vi "Init Module.vi"(8 "error in (no error)":errorcluster, 11 "Singleton Module Admin in":refnum<class "Delacor_lib_QMH_Module Admin.lvclass">) -> (0 "error out":errorcluster, 2 "DBModule Request Events":T1, 3 "Singleton Module Admin out":refnum<class "Delacor_lib_QMH_Module Admin.lvclass">)   [LabVIEW 2022 SP3, in "DBModule.lvlib"]
doc: "Initialize the module by creating Broadcast Events, Request Events, and synchronization rendezvous.\n____\nHAMPEL SOFTWARE ENGINEERING v2.6.0 (2023-12-19 10:54)"
uses:
  DBModule.lvlib
  <vilib>/Delacor/Delacor QMH/Libraries/Module Admin_class/Delacor_lib_QMH_Module Admin.lvclass
  Request Events--cluster.ctl
  Stop Argument--cluster.ctl
  Show Panel Argument--cluster.ctl
  Hide Panel Argument--cluster.ctl
  Get Module Execution Status Argument--cluster.ctl
  Show Diagram Argument--cluster.ctl
  Configure Argument--cluster.ctl
  Prepare Argument--cluster.ctl
  Request UI Display Argument--cluster.ctl
  Libraries/hse-libraries/Source/hse-dqmh/Controls/Module Display Scenarios.ctl
  Request UI Display (Reply Payload)--cluster.ctl
  Start and Configure DB_Connector Argument--cluster.ctl
  Libraries/hse-libraries/Source/hse-dqmh/hse-dqmh.lvlib
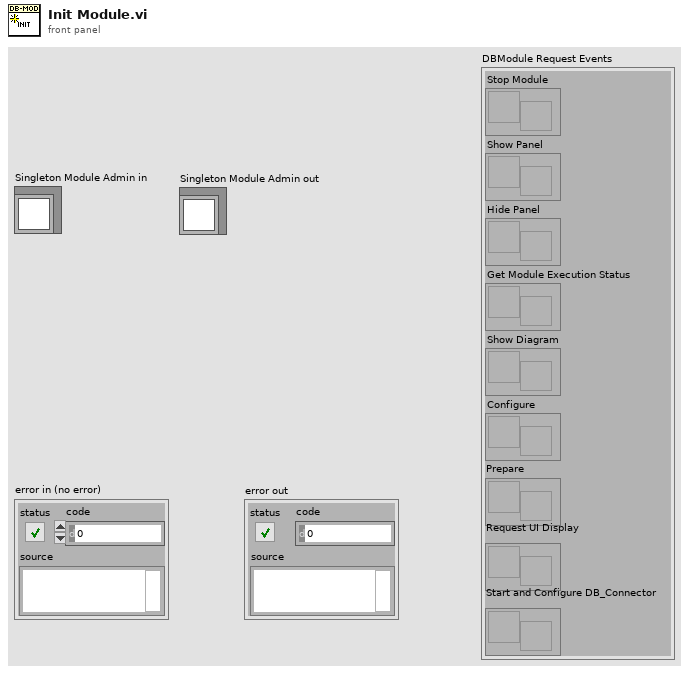
[diagram p1: front panel]
types:
  T1 = typedef "DBModule.lvlib/Request Events--cluster.ctl" = cluster{"Stop Module":refnum<user-event>, "Show Panel":refnum<user-event>, "Hide Panel":refnum<user-event>, "Get Module Execution Status":refnum<user-event>, "Show Diagram":refnum<user-event>, "Configure":refnum<user-event>, "Prepare":refnum<user-event>, "Request UI Display":refnum<user-event>, "Start and Configure DB_Connector":refnum<user-event>}
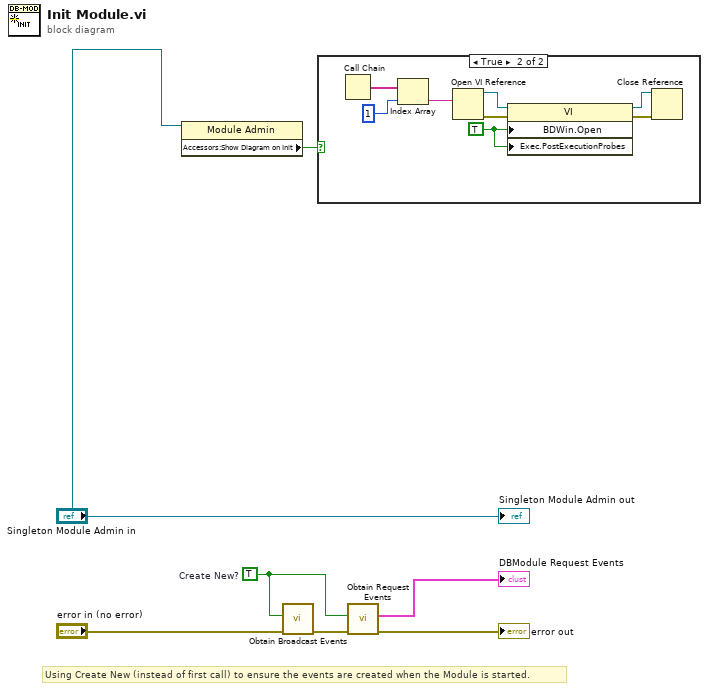
[diagram p0: block diagram]
diagram:
  w4 = TRUE  # Create New?
  # "Using Create New (instead of first call) to ensure the events are created when the Module is started."
  n1 = property class="Module Admin"(reference="Singleton Module Admin in") -> ("Accessors:Show Diagram on Init"=w1:bool)  [unwired: 1 in, 2 out]
  n2 = call "Obtain Broadcast Events.vi"("error in (no error)"="error in (no error)", "Create New? (F)"=w4) -> ("error out"=w7:errorcluster)  [unwired: 8 in, 1 out]
  n3 = case shown="True" w1 {
    frame False {
    }
    frame True {
      w11 = TRUE ("Block Diagram Window:Open")
      n4 = Call Chain() -> (call chain=w15:string[])
      n5 = Index Array(array=w15, index=1) -> (element=w8:string)
      n6 = Open VI Reference(vi path=w8) -> (vi reference=w12:refnum<vi>, error out=w13:errorcluster)  [unwired: 5 in]
      n7 = property class="VI"(reference=w12, error in=w13, "BDWin.Open"=w11, "Exec.PostExecutionProbes"=w11) -> (reference out=w9:refnum<vi>, error out=w10:errorcluster)
      n8 = Close Reference(reference=w9, error in (no error)=w10) -> ()  [unwired: 1 out]
    }
  }
  n9 = call "Obtain Request Events.vi"("error in (no error)"=w7, "Create New? (F)"=w4) -> ("error out"=→"error out":errorcluster, "DBModule Request Events"=→"DBModule Request Events":T1)  [unwired: 8 in]
  "Singleton Module Admin out" <- "Singleton Module Admin in"
